vi "LED2015 Ctlr Cmds.vi"(0 "VISA session":refnum<visa-resource-name>="COM11", 5 "Intensity":dbl(knob) min=0.0 max=100.0 step=1e-05 scale=0.0..100.0, 7 "High Gain":bool, 11 "error in (no error)":errorcluster) -> (4 "VISA session out":refnum<visa-resource-name>, 6 "Bytes at Port":u8, 8 "Response":string, 10 "Bytes Read":u8, 14 "High Gain":bool, 15 "error out":errorcluster)   [LabVIEW 2010]
uses:
  <vilib>/Instr/_visa.llb/VISA Flush IO Buffer Mask.ctl
  <vilib>/Instr/_visa.llb/VISA Configure Serial Port (Instr).vi
panel:
  out "Write Data (string)":string
  out "3 Byte Command":u8[](array[numeric]) format="%02x"
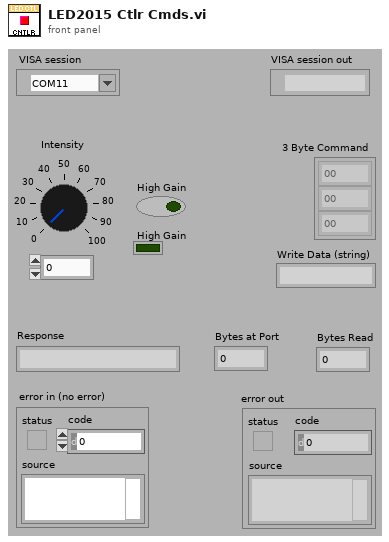
[diagram p1: front panel]
types:
  T1 = typedef "VISA Flush IO Buffer Mask.ctl" = u16
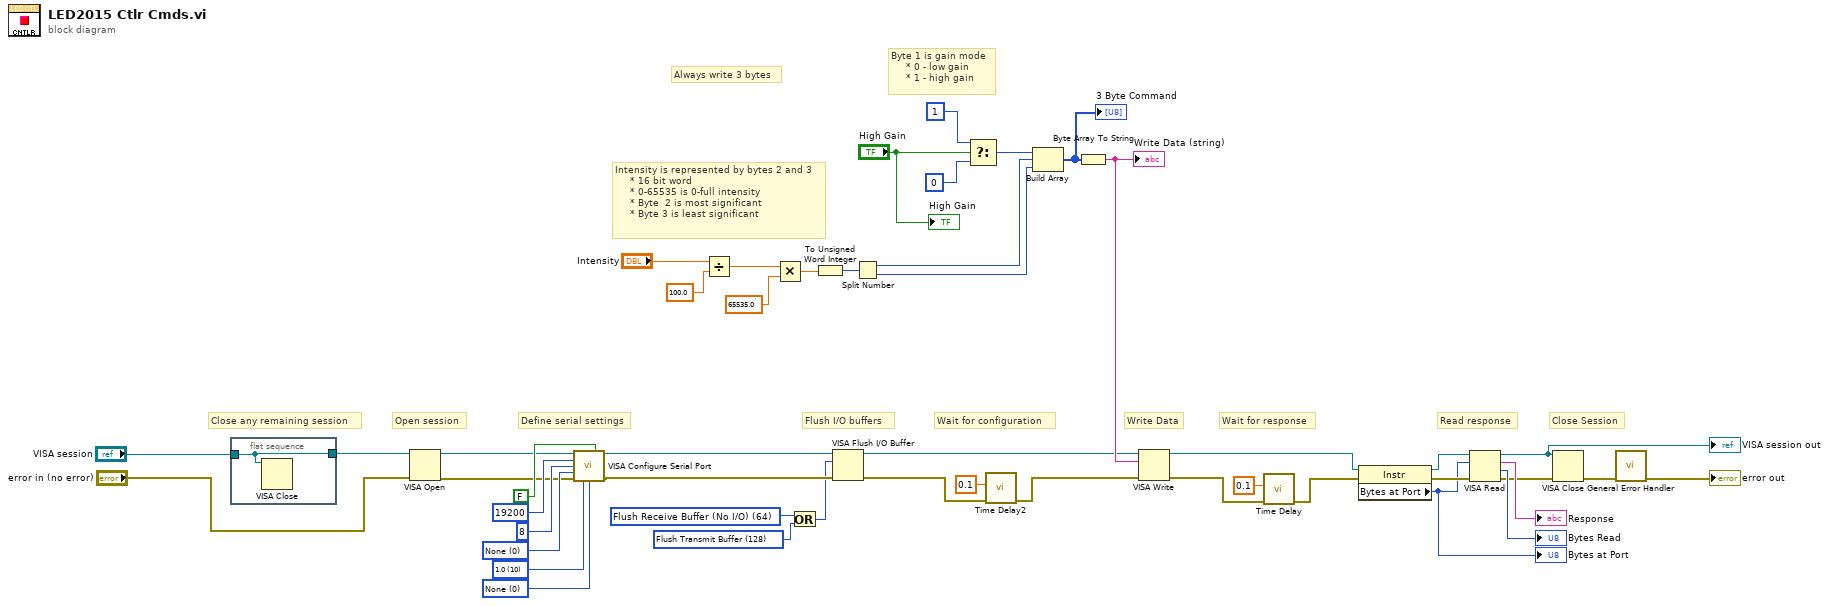
[diagram p0: block diagram]
diagram:
  w7 = T1 128 items=["Flush Receive Buffer"=16, "Write Transmit Buffer to Device"=32, "Flush Receive Buffer (No I/O)"=64, "Flush Transmit Buffer"=128] ("y")
  w8 = T1 64 items=["Flush Receive Buffer"=16, "Write Transmit Buffer to Device"=32, "Flush Receive Buffer (No I/O)"=64, "Flush Transmit Buffer"=128] ("Mask")
  w21 = u16 0 items=["None", "XON/XOFF", "RTS/CTS", "XON/XOFF & RTS/CTS", "DTR/DSR", "XON/XOFF & DTR/DSR"] ("Serial Settings:Flow Control")
  w20 = u16 10 items=["1.0"=10, "1.5"=15, "2.0"=20] ("Serial Settings:Stop Bits")
  w19 = u16 0 items=["None", "Odd", "Even", "Mark", "Space"] ("Serial Settings:Parity")
  # "Close Session"
  # "Close any remaining session"
  # "Wait for configuration"
  # "Open session"
  # "Define serial settings"
  # "Flush I/O buffers"
  # "Wait for response"
  # "Read response"
  # "Write Data"
  # "Always write 3 bytes"
  # "Byte 1 is gain mode\n     * 0 - low gain\n     * 1 - high gain"
  # "Intensity is represented by bytes 2 and 3\n     * 16 bit word\n     * 0-65535 is 0-full intensity\n     * Byte  2 is most significant\n     * Byte 3 is least significant"
  n1 = flat-sequence {
    tunnel: [w48] -> w14
    tunnel: "VISA session" -> [w48]
    frame #0 {
      n2 = VISA Close(VISA resource name=w48) -> ()  [unwired: 1 in, 1 out]
    }
  }
  n3 = VISA Open(error in (no error)="error in (no error)", VISA resource name=w14) -> (VISA resource name=w15:refnum<visa-resource-name>, error out=w16:errorcluster)  [unwired: 3 in]
  n4 = call-poly "VISA Configure Serial Port"("VISA resource name"=w15, "Enable Termination\nChar (T)"=FALSE ("Message Based Settings:Termination Character Enable"), "baud rate (9600)"=u32 19200 ("Serial Settings:Baud Rate"), "data bits (8)"=u16 8 ("Serial Settings:Data Bits"), "parity (0:none)"=w19, "error in (no error)"=w16, "stop bits (10: 1 bit)"=w20, "flow control (0:none)"=w21) -> ("VISA resource name out"=w9:refnum<visa-resource-name>, "error out"=w13:errorcluster)  [unwired: 6 in]
  n5 = Divide(x="Intensity", y=100.0) -> (x/y=w27:dbl)
  n6 = Multiply(x=w27, y=65535.0) -> (x*y=w28:dbl)
  n7 = Or(x=w8, y=w7) -> (x .or. y?=w6:T1)
  n8 = To Unsigned Word Integer(number=w28) -> (unsigned 16bit integer=w39:u16)
  n9 = VISA Flush I/O Buffer(VISA resource name=w9, mask (16)=w6, error in (no error)=w13) -> (VISA resource name out=w23:refnum<visa-resource-name>, error out=w10:errorcluster)
  n10 = Split Number(x=w39) -> (hi(x)=w26:u8, lo(x)=w5:u8)
  n11 = Select(t=u8 1 ("High Gain"), s="High Gain", f=u8 0 ("Low Gain")) -> (s? t:f=w4:u8)
  n12 = call "Time Delay2"("error in (no error)"=w10, "Delay Time (s)"=0.1) -> ("error out"=w11:errorcluster)  [unwired: 9 in]
  n13 = Build Array(w4, w26, w5) -> (w29:u8[])
  "3 Byte Command" <- w29
  n14 = Byte Array To String(unsigned byte array=w29) -> (string=w24:string)
  "Write Data (string)" <- w24
  n15 = VISA Write(VISA resource name=w23, write buffer=w24, error in (no error)=w11) -> (VISA resource name out=w35:refnum<visa-resource-name>, error out=w37:errorcluster)  [unwired: 1 out]
  n16 = call "Time Delay"("error in (no error)"=w37, "Delay Time (s)"=0.1) -> ("error out"=w36:errorcluster)  [unwired: 9 in]
  n17 = property class="Instr"(reference=w35, error in=w36) -> (reference out=w44:refnum<visa-resource-name>, error out=w43:errorcluster, "Bytes at Port"=w42:u32)
  "Bytes at Port" <- w42
  n18 = VISA Read(VISA resource name=w44, byte count=w42, error in (no error)=w43) -> (VISA resource name out=w1:refnum<visa-resource-name>, read buffer=→"Response":string, return count=→"Bytes Read":u32, error out=w3:errorcluster)
  "VISA session out" <- w1
  n19 = VISA Close(VISA resource name=w1, error in (no error)=w3) -> (error out=w45:errorcluster)
  n20 = call <vilib>:"General Error Handler.vi"("error in (no error)"=w45) -> ("error out"=→"error out":errorcluster)  [unwired: 10 in, 4 out]
  "High Gain" <- "High Gain"
